vi "Message_Init.vi"(8 "error in (no error)":errorcluster caption="错误输入（无错误）", 10 "根路径":path, 11 "文本框引用_输入":refnum<vi>) -> (0 "error out":errorcluster caption="错误输出", 3 "引用":string)   [LabVIEW 2012, in "Message.lvlib"]
uses:
  Message.lvlib
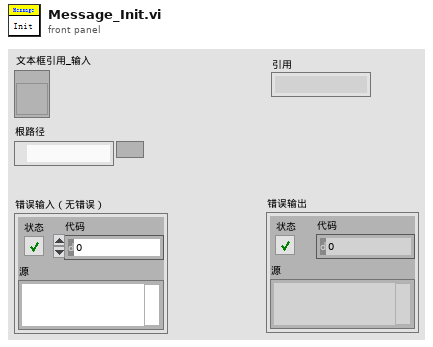
[diagram p1: front panel]
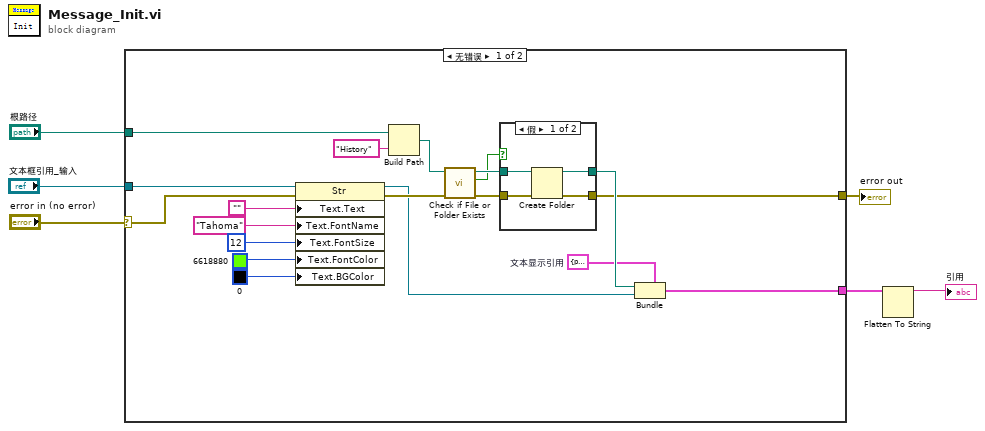
[diagram p0: block diagram]
diagram:
  n1 = case shown="无错误" "error in (no error)" {
    selector: "error in (no error)" -> [w19 w32]
    tunnel: [w9 w32] -> w5
    tunnel: "文本框引用_输入" -> [w25 _]
    tunnel: "根路径" -> [w18 _]
    tunnel: [w8 _] -> w2
    frame No Error {
      w7 = cluster{"LogPath":path, "信息框引用":refnum<vi>} {"LogPath"=path "", "信息框引用"=refnum}  # 文本显示引用
      n2 = property class="Str"(reference=w25, error in=w19, "Text.Text"="", "Text.FontName"="Tahoma" ("文本.字体:名称"), "Text.FontSize"=u32 12 ("文本.字体:字号"), "Text.FontColor"=u32 6618880, "Text.BGColor"=u32 0) -> (reference out=w10:refnum<vi>, error out=w16:errorcluster)
      n3 = Build Path(base path=w18, name or relative path="History" ("名称或相对路径")) -> (appended path=w15:path)
      n4 = call <vilib>:"Check if File or Folder Exists.vi"("error in (no error)"=w16, "path"=w15) -> ("error out"=w12:errorcluster, "file or folder exists?"=w13:bool, "dup path"=w14:path)  [unwired: 7 in]
      n5 = case shown="假" w13 {
        tunnel: w14 -> [w29 w30]
        tunnel: w12 -> [w28 w31]
        tunnel: [w27 w31] -> w9
        tunnel: [w26 w30] -> w11
        frame False {
          n6 = Create Folder(path (use dialog)=w29, error in=w28) -> (created path=w26:path, error out=w27:errorcluster)  [unwired: 1 in, 1 out]
        }
        frame True {
        }
      }
      n7 = Bundle(cluster=w7, "LogPath"=w11, "信息框引用"=w10) -> (w8:cluster{"LogPath":path, "信息框引用":refnum<vi>})
    }
    frame Error {
    }
  }
  "error out" <- w5
  n8 = Flatten To String(anything=w2) -> (data string=→"引用":string)  [unwired: 3 in, 2 out]
